vi "Judgment.vi"(7 "Name (\"\" to Use UUID)":string="Judgment") -> ()   [LabVIEW 2025]
doc: "Compact code template used to create a CSM module with a user interface. This template includes a user Event Structure for responding to user actions. The functionality of this template is identical to the CSM User Interface(UI) Module Template VI.\n\n\n> [!NOTE] <b>CSM Naming Rules</b>\n>\n> - CSM module name must be unique. Otherwise, CSM enters a `Critical Error` state.\n> - If the input module name is an empty string (\"\"), the system uses a UUID as the module name. Such a module is marked as standalone mode and does not appear in the module list.\n> - Worker Mode Rule: If the input module name ends with `#`, a worker mode node will be instantiated. Multiple worker mode nodes can form a worker mode module.\n> - Chain of Responsibility Mode Rule: If the input module name ends with `$` followed by a number, a chain of responsibility mode node will be instantiated. Multiple chain of responsibility mode nodes can form a chain of responsibility mode module.\n> - System-Level Module Rule: If the input module name starts with `.`, the module is a system-level module. Under default settings, such modules are not listed by the CSM - List Modules VI and are suitable for instantiating modules that run in the background.\n> - Submodule Rule: `.` is also allowed in a module name to separate the module name into multiple parts. CSM does not have strict rules for submodules. The `.` in the module name only marks the logical relationship between different modules. From an execution perspective, they are considered independent modules. The only difference is that you can obtain a list of logical submodules via the CSM - List Submodules VI.\n\n\n-- <b>Controls</b> --\n- <b>Name (\"\" to use UUID)</b>: CSM module name. Refer to <b>CSM Naming Rules</b> for module naming rules."
uses:
  <userlib>/_NEVSTOP/Communicable State Machine(CSM)/AdvanceAPI/CSM - Revert Arguments-Safe String.vi
  <userlib>/_NEVSTOP/Communicable State Machine(CSM)/_Shared/Trim Single-line Text.vi
  <userlib>/_NEVSTOP/Communicable State Machine(CSM)/AdvanceAPI/CSM - Break Down Multiple States String.vi
  <userlib>/_NEVSTOP/Communicable State Machine(CSM)/AdvanceAPI/CSM - Compact Multiple States.vi
  <userlib>/_NEVSTOP/Communicable State Machine(CSM)/AdvanceAPI/CSM - Make String Arguments Safe.vi
  <userlib>/_NEVSTOP/Communicable State Machine(CSM)/AdvanceAPI/CSM - Keywords.vi
  <userlib>/_NEVSTOP/Communicable State Machine(CSM)/Communicable State Machine.lvlib
panel:
  in  "Array":i32[](array[numeric])
  out "State History":string
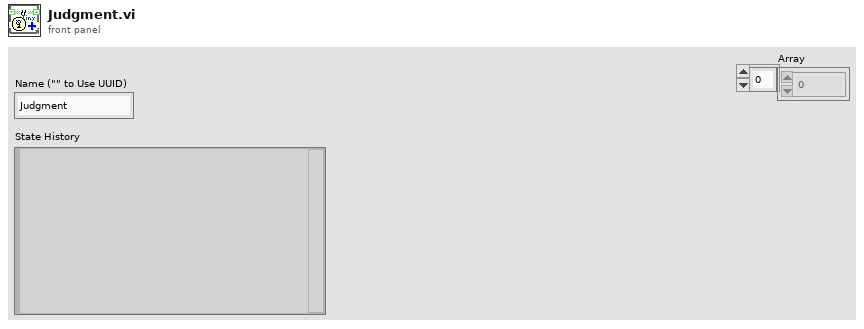
[diagram p1: front panel]
types:
  T1 = enum32{"Invalid", "Standard", "Closed", "Hidden", "Minimized", "Maximized"}
  T2 = enum32{"invalid app kind", "Development System", "Run Time System", "Student Edition", "Embedded LabVIEW", "Evaluation", "Custom"}
  T3 = typedef "Communicable State Machine.lvlib/_CSM_Response Source Message.ctl" = cluster{"‘State":string, "’Arguments":string, "’Error":errorcluster}
  T4 = cluster{"Current VI Reference":refnum<vi>, "Close Panel on Exit?":bool}
  T5 = cluster{"Core":cluster{"Current VI Reference":refnum<vi>, "Close Panel on Exit?":bool}, "T0":i64, "BeatInterval":i32, "NoteIndex":i32}
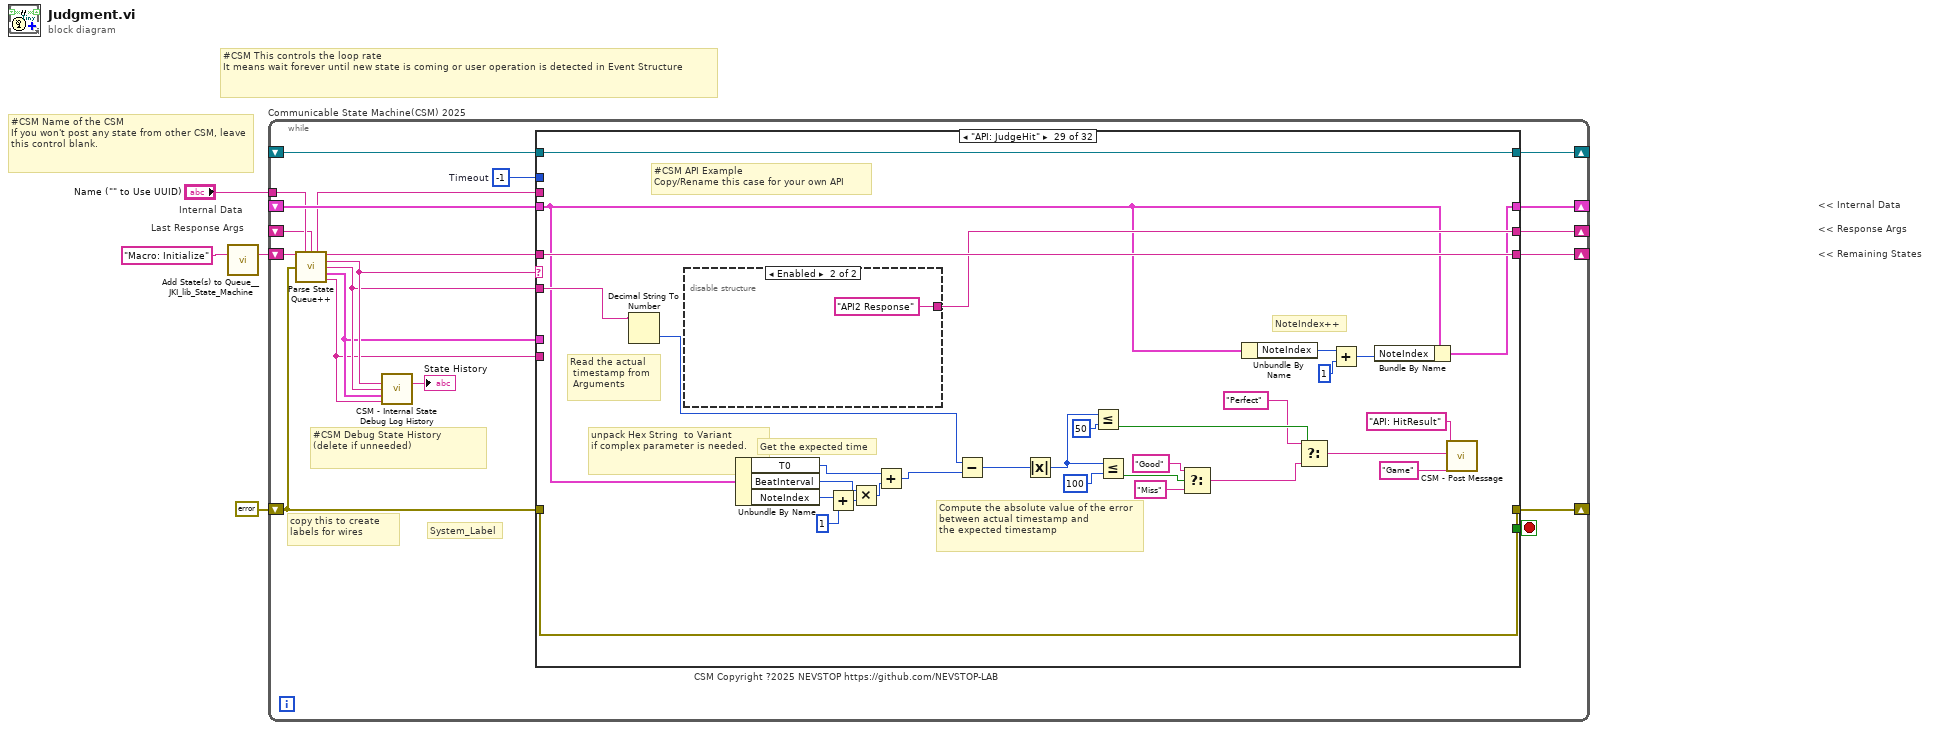
[diagram p0: block diagram]
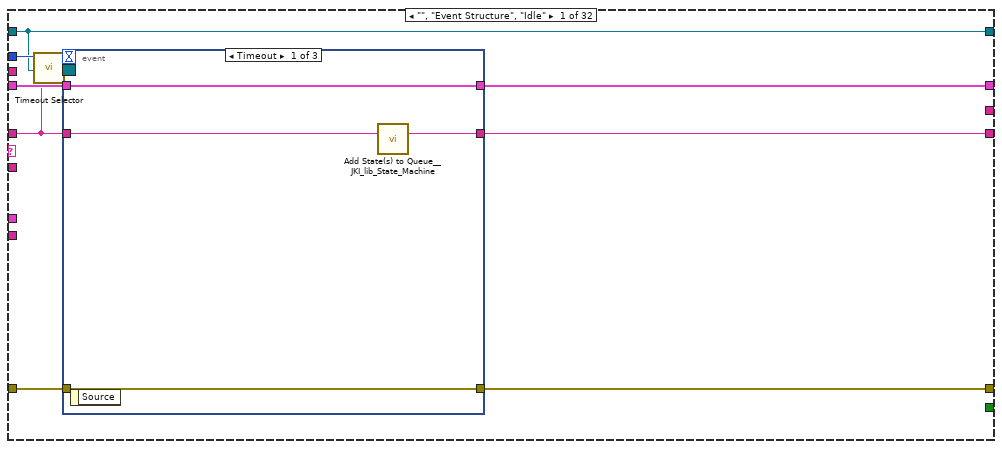
[diagram p2: hidden frame]
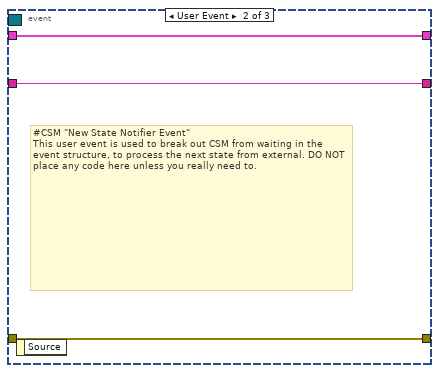
[diagram p3: hidden frame]
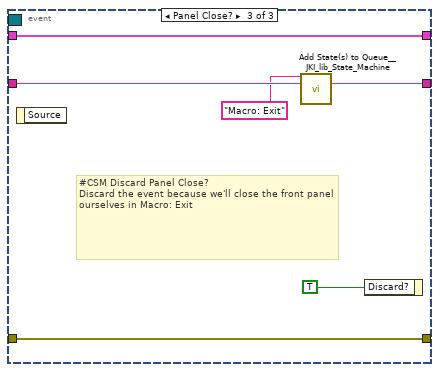
[diagram p4: hidden frame]
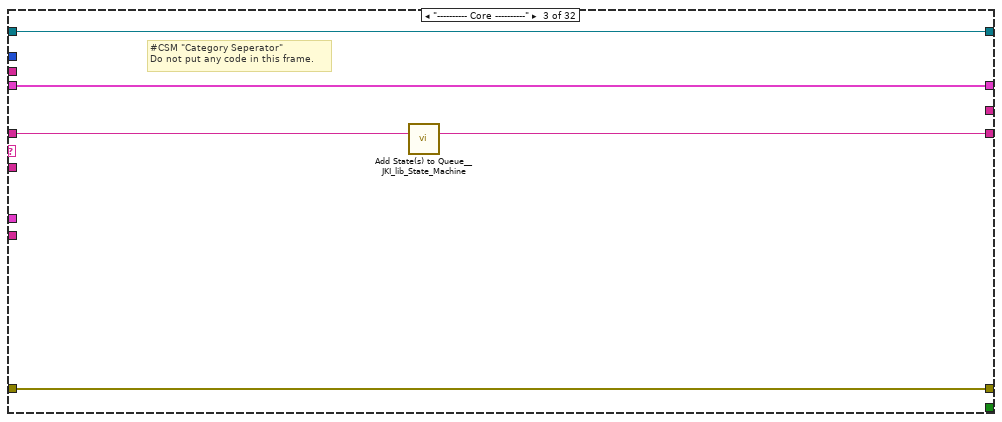
[diagram p6: hidden frame]
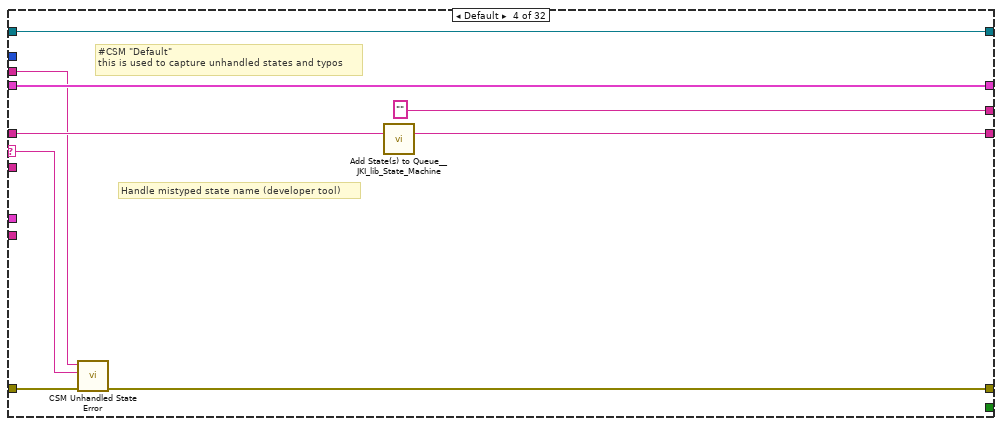
[diagram p7: hidden frame]
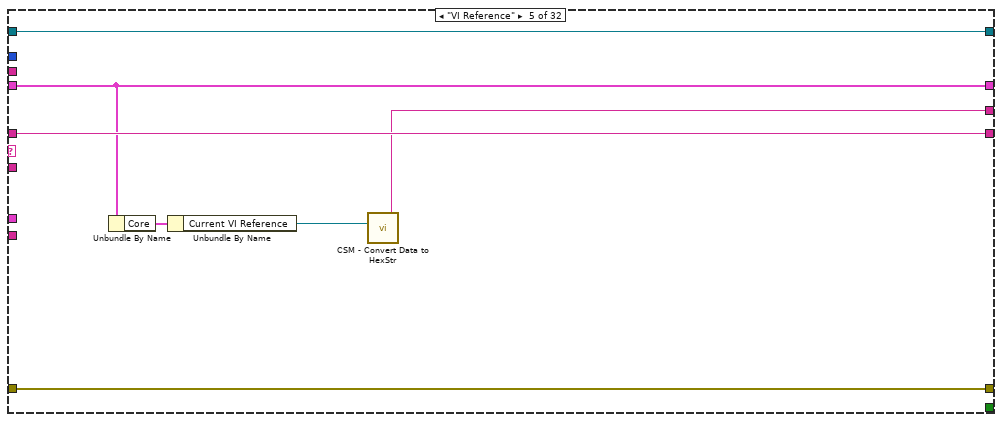
[diagram p8: hidden frame]
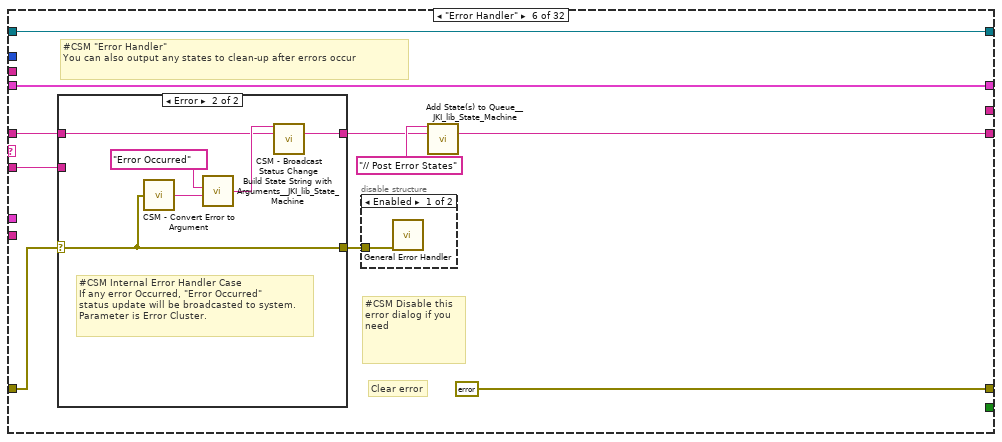
[diagram p9: hidden frame]
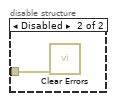
[diagram p10: hidden frame]
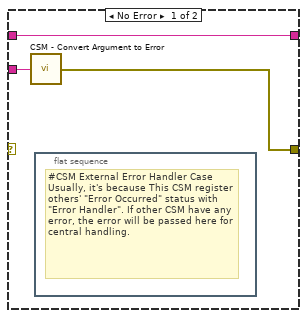
[diagram p11: hidden frame]
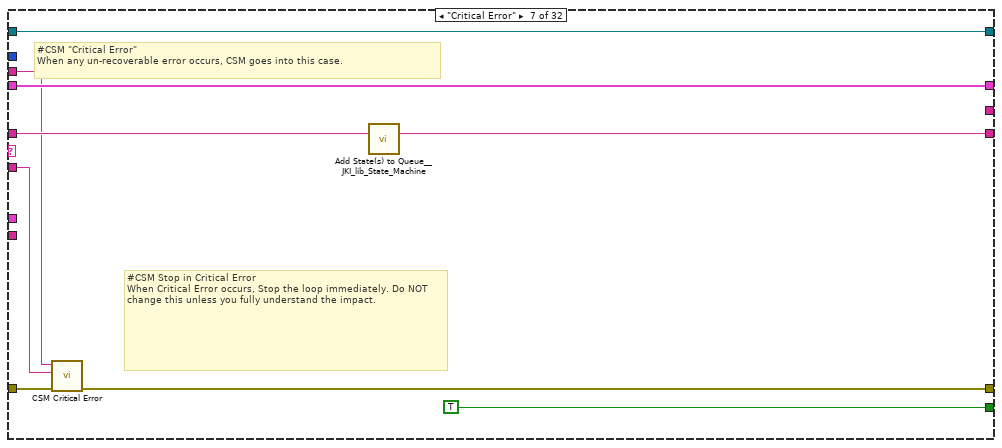
[diagram p12: hidden frame]
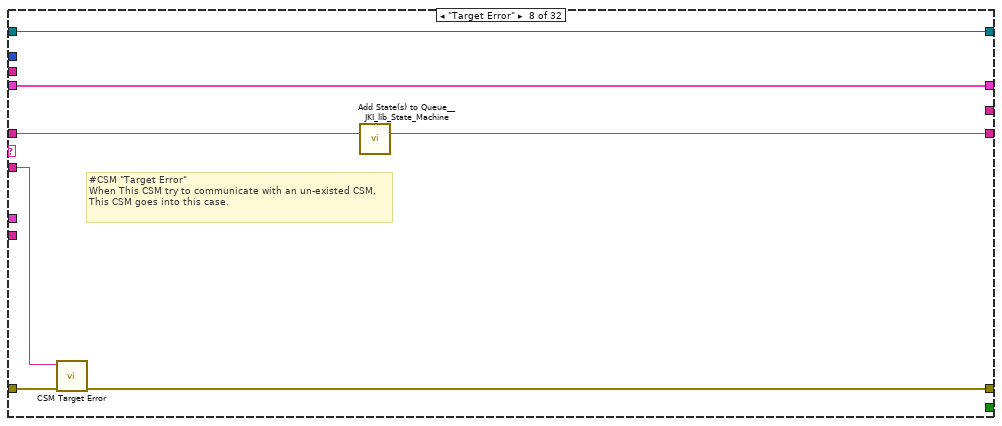
[diagram p13: hidden frame]
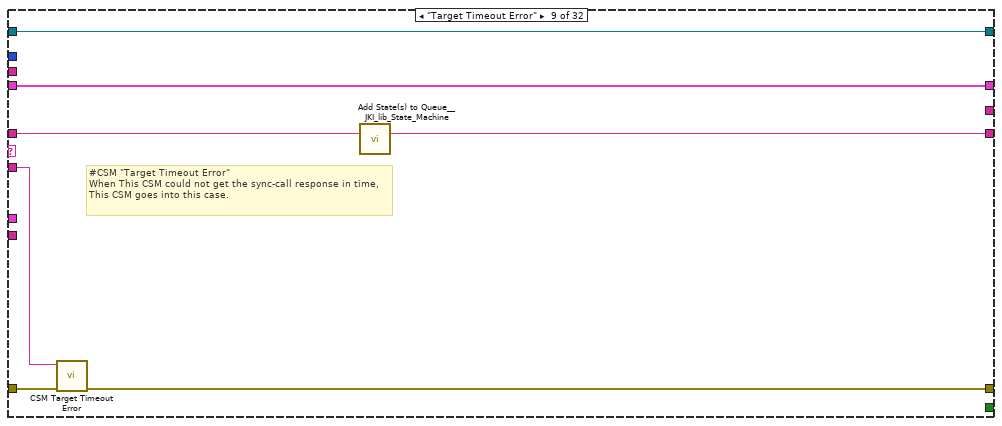
[diagram p14: hidden frame]
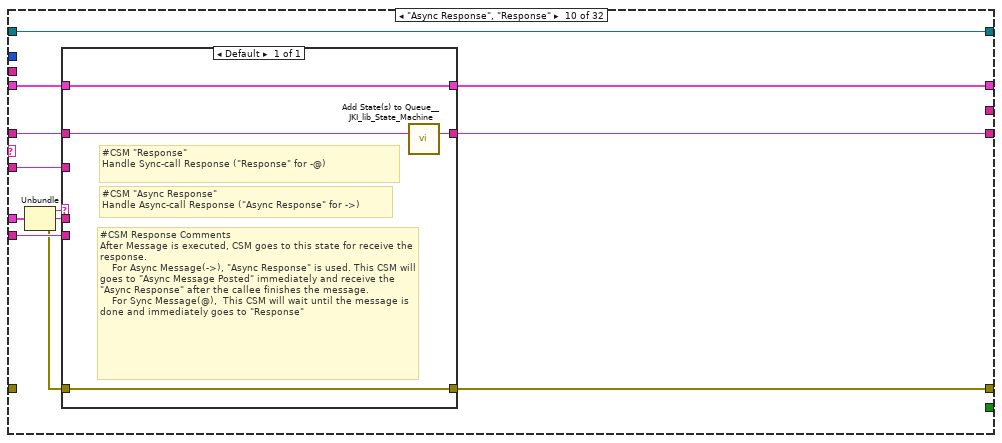
[diagram p15: hidden frame]
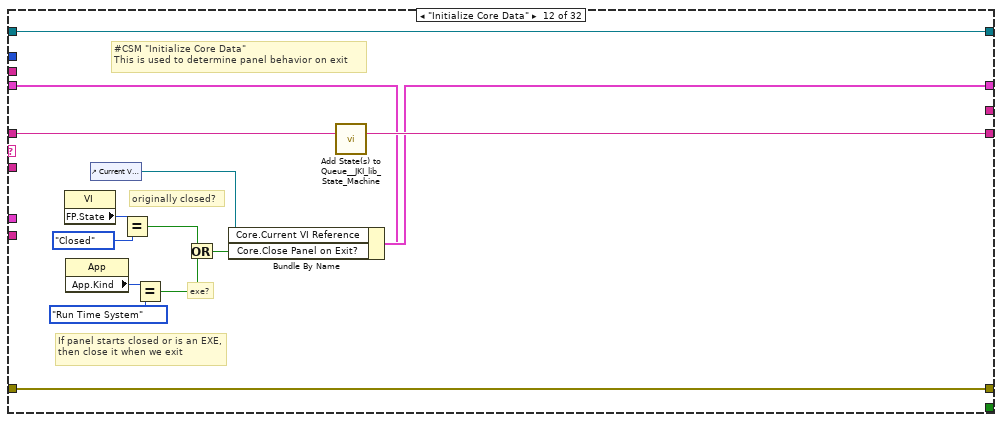
[diagram p17: hidden frame]
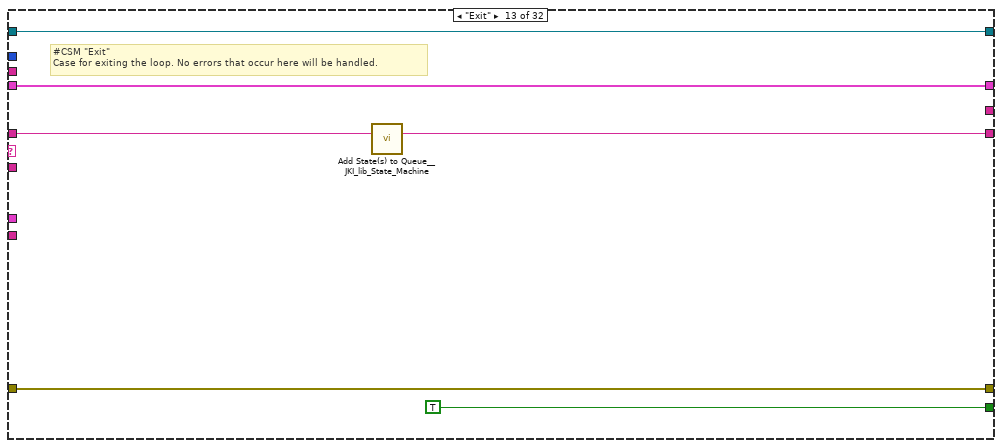
[diagram p18: hidden frame]
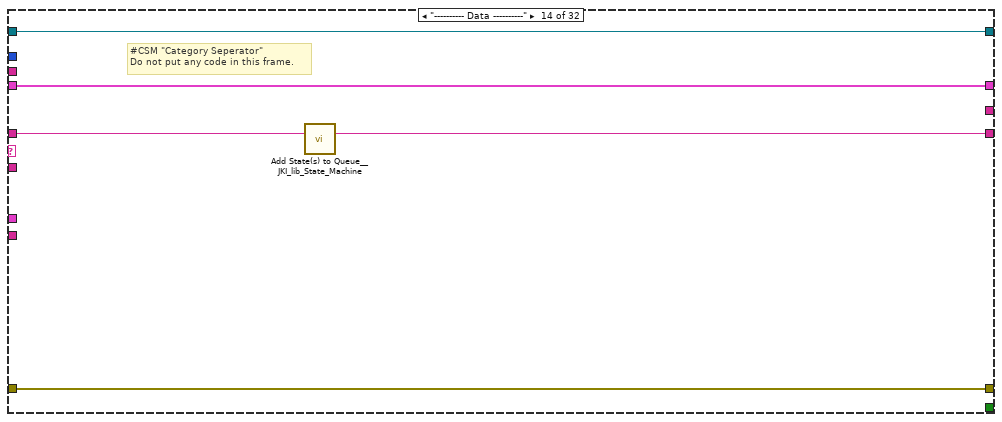
[diagram p19: hidden frame]
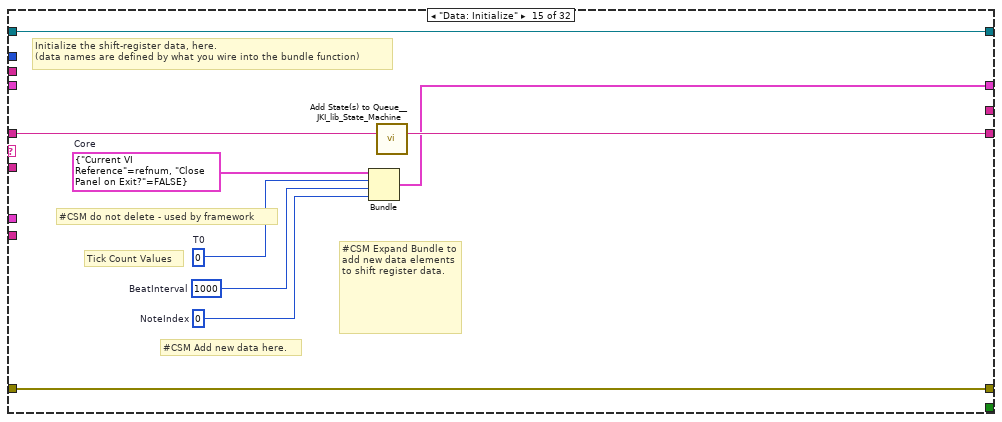
[diagram p20: hidden frame]
diagram:
  # "Last Response Args"
  # "Internal Data"
  # "#CSM Name of the CSM\nIf you won't post any state from other CSM, leave this control blank."
  # "#CSM This controls the loop rate\nIt means wait forever until new state is coming or user operation is detected in Event Structure"
  # "<< Internal Data"
  # "<< Response Args"
  # "<< Remaining States"
  n1 = call <vilib>:"Add State(s) to Queue__JKI_lib_State_Machine.vi"("State(s) in (\"\")"="Macro: Initialize" ("Init State(\"Macro: Initialize\")")) -> ("States Out"=w4:string)  [unwired: 14 in]
  n2 = while "Communicable State Machine(CSM) 2025" {
    shift-right: [w19] -> _
    shift-left: _ -> [w18]
    shift-right: [w22] -> _
    shift-left: errorcluster {"status"=FALSE, "code"=0, "source"=""} ("error out") -> [w16]
    shift-right: [w21] -> _
    shift-left: w4 -> [w23]
    tunnel: "Name (\"\" to Use UUID)" -> [w12]
    shift-right: [w15] -> _
    shift-left: _ -> [w6]
    shift-right: [w14] -> _
    shift-left: _ -> [w13]
    stop <- w20 stop-if-true
    w17 = -1  # Timeout
    # "#CSM Debug State History\n(delete if unneeded)"
    # "copy this to create labels for wires"
    # "System_Label"
    # "CSM Copyright ?2025 NEVSTOP https://github.com/NEVSTOP-LAB"
    n3 = call <userlib>:"Parse State Queue++.vi"("State Queue"=w23, "Name (\"\" to Use UUID)"=w12, "Response Arguments"=w6, "Previous Error"=w16) -> ("Name Used"=w7:string, "Remaining States"=w24:string, "Current State"=w11:string, "Arguments"=w10:string, "Additional Information"=w9:T3, "Source CSM"=w8:string)  [unwired: 6 in]
    n4 = call <userlib>:"CSM - Internal State Debug Log History.vi"("State"=w11, "Arguments (\"\")"=w10, ">> Response Source Message >>"=w9, "Source (\"\")"=w8) -> ("Debug Log"=→"State History":string)  [unwired: 11 in]
    n5 = case shown="\"API: JudgeHit\"" w11 {
      selector: w11 -> [_ _ _ w58 _ _ _ _ _ _ _ _ _ _ _ _ _ _ _ _ _ _ _ _ _ _ _ _ _ _ _ _]
      tunnel: w24 -> [w25 w49 w55 w63 w70 w76 w99 w105 w112 w121 w134 w149 w155 w160 w169 w176 w181 w188 w192 w198 w203 w210 w226 w296 w302 w314 w317 w333 w364 w372 w377 w382]
      tunnel: w10 -> [_ _ _ _ _ w75 w94 w104 w111 w120 _ _ _ _ _ _ _ _ _ _ _ w205 w220 _ _ _ _ w330 w361 _ _ _]
      tunnel: w18 -> [w32 w48 w52 w61 w69 w80 w100 w107 w114 w123 w133 w142 w153 w157 _ w171 w178 w187 w191 w195 w201 w208 w222 w293 w299 w311 w316 w324 w339 w369 w374 w379]
      tunnel: [w31 w50 w53 w56 w71 errorcluster {"status"=FALSE, "code"=0, "source"=""} ("error out") w95 w102 w109 w126 w135 w146 w152 w158 w166 w172 w179 w182 w190 w196 w200 w206 w223 w294 w300 w312 w318 w334 w365 w370 w375 w380] -> w22
      tunnel: w16 -> [w30 w50 w53 w64 w71 w77 w101 w103 w110 _ w135 w146 w152 w158 w166 w173 w179 _ w193 w196 w200 w207 w224 w294 w300 w312 w318 w334 w365 w370 w375 w380]
      tunnel: [w33 w49 w54 w62 w70 w72 w98 w108 w115 w122 w134 w148 w154 w159 w168 w175 w180 w188 w192 w197 w202 w209 w225 w295 w301 w313 w317 w333 w364 w371 w376 w381] -> w21
      tunnel: [_ _ _ _ _ _ TRUE _ _ _ _ _ TRUE _ _ _ _ _ _ _ _ _ _ _ _ _ _ _ _ _ _ _] -> w20
      tunnel: [w29 w48 w52 w61 w69 w80 w100 w107 w114 w124 w133 w147 w153 w157 w167 w171 w178 w187 w191 w195 w201 w208 w222 w293 w299 w311 w316 w320 w338 w369 w374 w379] -> w19
      tunnel: w17 -> [w28 _ _ _ _ _ _ _ _ _ _ _ _ _ _ _ _ _ _ _ _ _ _ _ _ _ _ _ _ _ _ _]
      tunnel: w8 -> [_ _ _ _ _ _ _ _ _ w118 _ _ _ _ _ _ _ _ _ _ _ _ _ _ _ _ _ _ _ _ _ _]
      tunnel: w9 -> [_ _ _ _ _ _ _ _ _ w125 _ _ _ _ _ _ _ _ _ _ _ _ _ _ _ _ _ _ _ _ _ _]
      tunnel: [_ _ _ "" w65 _ _ _ _ _ _ _ _ _ _ _ _ _ _ _ _ _ _ _ _ _ _ "API1 Response" w362 _ _ _] -> w15
      tunnel: [w27 w47 w51 w59 w68 w79 w96 w106 w113 w127 w132 w136 w150 w156 w164 w170 w177 w186 w189 w194 w199 w204 w219 w292 w297 w304 w315 w332 w363 w368 w373 w378] -> w14
      tunnel: w13 -> [w27 w47 w51 w59 w68 w79 w96 w106 w113 w127 w132 w136 w150 w156 w164 w170 w177 _ w189 w194 w199 w204 w219 w292 w297 w304 w315 w332 w363 w368 w373 w378]
      tunnel: w7 -> [_ _ _ w57 _ _ w93 _ _ _ _ _ _ _ _ _ _ w185 _ _ _ _ _ _ _ _ _ _ _ _ _ _]
      frame "", "Event Structure", "Idle" {
        n6 = call <userlib>:"Timeout Selector.vi"("Remaining States"=w25, "Timeout Expected"=w28) -> ("Timeout"=w26:i32)  [unwired: 5 in]
        n7 = event shown="[0] Timeout" {
          selector: w27 -> [_ _ _]
          dyn-events: _ -> [_ _ _]
          timeout: w26 -> [_ _ _]
          tunnel: w25 -> [w37 w39 w46]
          tunnel: [w36 w39 w45] -> w33
          tunnel: w32 -> [w34 w40 w43]
          tunnel: [w35 w38 w44] -> w31
          tunnel: w30 -> [w35 w38 w44]
          tunnel: [w34 w40 w43] -> w29
          event Timeout {
            n8 = event-data() -> ()  [unwired: 1 in, 1 out]
            n9 = call <vilib>:"Add State(s) to Queue__JKI_lib_State_Machine.vi"("State(s) in (\"\")"=w37) -> ("States Out"=w36:string)  [unwired: 14 in]
          }
          event User Event {
            # "#CSM \"New State Notifier Event\"\nThis user event is used to break out CSM from waiting in the event structure, to process the next state from external. DO NOT place any code here unless you really need to."
            n10 = event-data() -> ()  [unwired: 1 in, 1 out]
          }
          event Panel Close? {
            # "#CSM Discard Panel Close?\nDiscard the event because we'll close the front panel ourselves in Macro: Exit"
            n11 = event-data() -> ()  [unwired: 1 in, 1 out]
            n12 = call <vilib>:"Add State(s) to Queue__JKI_lib_State_Machine.vi"("State(s) in Front (\"\")"="Macro: Exit", "State(s) in (\"\")"=w46) -> ("States Out"=w45:string)  [unwired: 13 in]
            n13 = event-data("Discard?"=TRUE) -> ()  [unwired: 1 in, 1 out]
          }
        }
      }
      frame "CSM Documentation" {
        # "#CSM README FIRST\n\nCommunicable State Machine(CSM) is a LabVIEW application framework that builds upon JKI State Machine(JKISM). It follows the pattern of JKISM and extends the keywords to describe message communication between modules, including concepts such as Sync-Message, Async-Message, Subscription/Unsubscription of status - essential elements for creating reusable code modules. For more information, please visit the CSM wiki: https://nevstop-lab.github.io/CSM-Wiki/\n\nFor instructions on JKI State Machine, visit: http://jki.net/state-machine/\nFor information about CSM, visit: https://github.com/NEVSTOP-LAB"
        # "#CSM \"Documentation\"\nCase for holding CSM Documenation"
      }
      frame "---------- Core ----------" {
        # "#CSM \"Category Seperator\"\nDo not put any code in this frame."
        n14 = call <vilib>:"Add State(s) to Queue__JKI_lib_State_Machine.vi"("State(s) in (\"\")"=w55) -> ("States Out"=w54:string)  [unwired: 14 in]
      }
      frame Default {
        # "#CSM \"Default\"\nthis is used to capture unhandled states and typos"
        # "Handle mistyped state name (developer tool)"
        n15 = call <userlib>:"CSM Unhandled State Error.vi"("error in (no error)"=w64, "Undefined State"=w58, "CSM Name"=w57) -> ("error out"=w56:errorcluster)  [unwired: 8 in]
        n16 = call <vilib>:"Add State(s) to Queue__JKI_lib_State_Machine.vi"("State(s) in (\"\")"=w63) -> ("States Out"=w62:string)  [unwired: 14 in]
      }
      frame "VI Reference" {
        n17 = Unbundle By Name(w69) -> ("Core"=w67:T4)
        n18 = Unbundle By Name(w67) -> ("Current VI Reference"=w66:refnum<vi>)
        n19 = call <userlib>:"CSM - Convert Data to HexStr.vi"("Variant"=w66) -> ("HEX String (0-9,A-F)"=w65:string)  [unwired: 8 in]
      }
      frame "Error Handler" {
        # "#CSM Disable this error dialog if you need"
        # "#CSM \"Error Handler\"\nYou can also output any states to clean-up after errors occur"
        # "Clear error"
        n20 = case shown="Error" w77 {
          selector: w77 -> [_ w87]
          tunnel: [w86 w89] -> w73
          tunnel: w76 -> [w86 w88]
          tunnel: w75 -> [w85 _]
          tunnel: [w84 w87] -> w78
          frame No Error {
            n21 = call <userlib>:"CSM - Convert Argument to Error.vi"("Argument"=w85) -> ("Error"=w84:errorcluster)  [unwired: 4 in]
            n22 = flat-sequence {
              frame #0 {
                # "#CSM External Error Handler Case\nUsually, it's because This CSM register others' \"Error Occurred\" status with \"Error Handler\". If other CSM have any error, the error will be passed here for central handling."
              }
            }
          }
          frame Error {
            # "#CSM Internal Error Handler Case \nIf any error Occurred, \"Error Occurred\" \nstatus update will be broadcasted to system.\nParameter is Error Cluster."
            n23 = call <userlib>:"CSM - Convert Error to Argument.vi"("Error"=w87) -> ("Argument"=w91:string)  [unwired: 4 in]
            n24 = call <vilib>:"Build State String with Arguments__JKI_lib_State_Machine.vi"("Arguments (\"\")"=w91, "State"="Error Occurred" ("Status with Arguments")) -> ("State with Arguments"=w90:string)  [unwired: 4 in]
            n25 = call <userlib>:"CSM - Broadcast Status Change.vi"("Status With Arguments"=w90, "State Queue"=w88) -> ("Remaining States"=w89:string)  [unwired: 13 in]
          }
        }
        n26 = disable-structure shown="Enabled" {
          disable-tunnel: w78 -> [w82 w83]
          frame Enabled {
            n27 = call <vilib>:"General Error Handler.vi"("error in (no error)"=w82) -> ()  [unwired: 10 in, 5 out]
          }
          frame Disabled {
            n28 = call <vilib>:"Clear Errors.vi"("error in (no error)"=w83) -> ()  [unwired: 5 in, 2 out]
          }
        }
        n29 = call <vilib>:"Add State(s) to Queue__JKI_lib_State_Machine.vi"("State(s) in Front (\"\")"="// Post Error States", "State(s) in (\"\")"=w73) -> ("States Out"=w72:string)  [unwired: 13 in]
      }
      frame "Critical Error" {
        # "#CSM Stop in Critical Error\nWhen Critical Error occurs, Stop the loop immediately. Do NOT change this unless you fully understand the impact."
        # "#CSM \"Critical Error\"\nWhen any un-recoverable error occurs, CSM goes into this case."
        n30 = call <userlib>:"CSM Critical Error.vi"("error in (no error)"=w101, "Arugments (As Reason)"=w94, "CSM Name"=w93) -> ("error out"=w95:errorcluster)  [unwired: 8 in]
        n31 = call <vilib>:"Add State(s) to Queue__JKI_lib_State_Machine.vi"("State(s) in (\"\")"=w99) -> ("States Out"=w98:string)  [unwired: 14 in]
      }
      frame "Target Error" {
        # "#CSM \"Target Error\"\nWhen This CSM try to communicate with an un-existed CSM, This CSM goes into this case."
        n32 = call <userlib>:"CSM Target Error.vi"("error in (no error)"=w103, "Arguments (As CSM Name)"=w104) -> ("error out"=w102:errorcluster)  [unwired: 9 in]
        n33 = call <vilib>:"Add State(s) to Queue__JKI_lib_State_Machine.vi"("State(s) in (\"\")"=w105) -> ("States Out"=w108:string)  [unwired: 14 in]
      }
      frame "Target Timeout Error" {
        # "#CSM \"Target Timeout Error\"\nWhen This CSM could not get the sync-call response in time, This CSM goes into this case."
        n34 = call <userlib>:"CSM Target Timeout Error.vi"("error in (no error)"=w110, "Arguments (As CSM Name)"=w111) -> ("error out"=w109:errorcluster)  [unwired: 9 in]
        n35 = call <vilib>:"Add State(s) to Queue__JKI_lib_State_Machine.vi"("State(s) in (\"\")"=w112) -> ("States Out"=w115:string)  [unwired: 14 in]
      }
      frame "Async Response", "Response" {
        n36 = Unbundle(w125) -> ("‘State"=w119:string, "’Arguments"=w117:string, "’Error"=w116:errorcluster)
        n37 = case shown="Default" w119 {
          tunnel: [w131] -> w126
          tunnel: w116 -> [w131]
          tunnel: [w130] -> w124
          tunnel: w123 -> [w130]
          tunnel: [w128] -> w122
          tunnel: w121 -> [w129]
          tunnel: w120 -> [_]
          tunnel: w118 -> [_]
          tunnel: w117 -> [_]
          frame Default {
            # "#CSM Response Comments\nAfter Message is executed, CSM goes to this state for receive the response.\n    For Async Message(->), \"Async Response\" is used. This CSM will goes to \"Async Message Posted\" immediately and receive the \"Async Response\" after the callee finishes the message.\n    For Sync Message(@),  This CSM will wait until the message is done and immediately goes to \"Response\""
            # "#CSM \"Async Response\"\nHandle Async-call Response (\"Async Response\" for ->)"
            # "#CSM \"Response\"\nHandle Sync-call Response (\"Response\" for -@)"
            n38 = call <vilib>:"Add State(s) to Queue__JKI_lib_State_Machine.vi"("State(s) in (\"\")"=w129) -> ("States Out"=w128:string)  [unwired: 14 in]
          }
        }
      }
      frame "Async Message Posted" {
        # "#CSM \"Async Message Posted\"\nAfter Async Message is posted (-> or ->| ), CSM goes to this state for post-action.\nYou can use Argument - State to tell which Async Message is called."
      }
      frame "Initialize Core Data" {
        # "#CSM \"Initialize Core Data\"\nThis is used to determine panel behavior on exit"
        # "originally closed?"
        # "exe?"
        # "If panel starts closed or is an EXE, then close it when we exit"
        n39 = property class="VI"() -> ("FP.State"=w139:T1)  [unwired: 2 in, 2 out]
        n40 = property class="App"() -> ("App.Kind"=w145:T2)  [unwired: 2 in, 2 out]
        n41 = control-ref of="Current VI Reference"() -> (w140:refnum<vi>)
        n42 = Equal?(x=w139, y=T1."Closed" ("Front Panel Window:State")) -> (x = y?=w137:bool)
        n43 = Equal?(x=w145, y=T2."Run Time System" ("Application:Kind")) -> (x = y?=w143:bool)
        n44 = Or(x=w137, y=w143) -> (x .or. y?=w141:bool)
        n45 = Bundle By Name(cluster=w142, "Core.Current VI Reference"=w140, "Core.Close Panel on Exit?"=w141) -> (w147:T5)
        n46 = call <vilib>:"Add State(s) to Queue__JKI_lib_State_Machine.vi"("State(s) in (\"\")"=w149) -> ("States Out"=w148:string)  [unwired: 14 in]
      }
      frame "Exit" {
        # "#CSM \"Exit\"\nCase for exiting the loop. No errors that occur here will be handled."
        n47 = call <vilib>:"Add State(s) to Queue__JKI_lib_State_Machine.vi"("State(s) in (\"\")"=w155) -> ("States Out"=w154:string)  [unwired: 14 in]
      }
      frame "---------- Data ----------" {
        # "#CSM \"Category Seperator\"\nDo not put any code in this frame."
        n48 = call <vilib>:"Add State(s) to Queue__JKI_lib_State_Machine.vi"("State(s) in (\"\")"=w160) -> ("States Out"=w159:string)  [unwired: 14 in]
      }
      frame "Data: Initialize" {
        w161 = 0  # NoteIndex
        w162 = 1000  # BeatInterval
        w163 = i64 0  # T0
        w165 = T4 {"Current VI Reference"=refnum, "Close Panel on Exit?"=FALSE}  # Core
        # "Tick Count Values"
        # "#CSM do not delete - used by framework"
        # "#CSM Expand Bundle to add new data elements to shift register data."
        # "#CSM Add new data here."
        # "Initialize the shift-register data, here.\n(data names are defined by what you wire into the bundle function)"
        n49 = Bundle("Core"=w165, "T0"=w163, "BeatInterval"=w162, "NoteIndex"=w161) -> (w167:T5)  [unwired: 1 in]
        n50 = call <vilib>:"Add State(s) to Queue__JKI_lib_State_Machine.vi"("State(s) in (\"\")"=w169) -> ("States Out"=w168:string)  [unwired: 14 in]
      }
      frame "Data: Cleanup" {
        # "Cleanup any data and references, here.\n(this is called automatically, by the Macro: Exit)"
        n51 = Unbundle By Name(w171) -> ("Core.Current VI Reference"=w174:refnum<vi>)
        n52 = Close Reference(reference=w174, error in (no error)=w173) -> (error out=w172:errorcluster)
        n53 = call <vilib>:"Add State(s) to Queue__JKI_lib_State_Machine.vi"("State(s) in (\"\")"=w176) -> ("States Out"=w175:string)  [unwired: 14 in]
      }
      frame "---------- Events ----------" {
        # "#CSM \"Category Seperator\"\nDo not put any code in this frame."
        n54 = call <vilib>:"Add State(s) to Queue__JKI_lib_State_Machine.vi"("State(s) in (\"\")"=w181) -> ("States Out"=w180:string)  [unwired: 14 in]
      }
      frame "Events: Register" {
        # "#CSM \"Events: Register\"\nRegister user event. New Message Event is registered to break CSM waiting in event structure by default."
        # "#CSM Register New Message Event\nRegister message event to break Waiting in Event structure."
        n55 = call <userlib>:"CSM - Get New State Notifier Event.vi"("Name (\"\" to Use UUID)"=w185) -> ("error out"=w183:errorcluster, "New State Notifier Event"=w184:refnum<user-event>)  [unwired: 9 in]
        n56 = register-events(error in=w183, w184) -> (reference out=w186:refnum<event-registration>, error out=w182:errorcluster)  [unwired: 1 in]
      }
      frame "Events: Unregister" {
        # "#CSM \"Events: Unregister\"\nUnregister user event."
        n57 = Unregister For Events(event registration refnum=w189, error in=w193) -> (error out=w190:errorcluster)
      }
      frame "---------- UI ----------" {
        # "#CSM \"Category Seperator\"\nDo not put any code in this frame."
        n58 = call <vilib>:"Add State(s) to Queue__JKI_lib_State_Machine.vi"("State(s) in (\"\")"=w198) -> ("States Out"=w197:string)  [unwired: 14 in]
      }
      frame "UI: Initialize" {
        # "#CSM \"UI: Initialize\"\nInitialize the User Interface, here.\n(this is called automatically, by the Macro: Init)"
        n59 = call <vilib>:"Add State(s) to Queue__JKI_lib_State_Machine.vi"("State(s) in (\"\")"=w203) -> ("States Out"=w202:string)  [unwired: 14 in]
      }
      frame "UI: Cursor Set" {
        # "#CSM \"UI: Cursor Set\"\nSet and Unset Cursor Busy.\n(Usage: \"UI: Cursor Set >> Busy|Idle\")"
        # "Argument"
        n60 = disable-structure shown="Default" {
          disable-tunnel: w207 -> [w213 w218]
          disable-tunnel: [w212 w218] -> w206
          disable-tunnel: w205 -> [w211 _]
          frame condition #0 (active) {
            n61 = case shown="\"Idle\", Default" w211 {
              tunnel: w213 -> [w215 w217]
              tunnel: [w214 w216] -> w212
              frame "Idle", Default {
                n62 = call <vilib>:"Unset Busy.vi"("error in (no error)"=w215) -> ("error out"=w214:errorcluster)  [unwired: 10 in]
              }
              frame "Busy" {
                n63 = call <vilib>:"Set Busy.vi"("error in (no error)"=w217) -> ("error out"=w216:errorcluster)  [unwired: 9 in, 1 out]
              }
            }
          }
          frame condition #1 {
          }
        }
        n64 = call <vilib>:"Add State(s) to Queue__JKI_lib_State_Machine.vi"("State(s) in (\"\")"=w210) -> ("States Out"=w209:string)  [unwired: 14 in]
      }
      frame "UI: Front Panel State" {
        # "#CSM \"UI: Front Panel State\"\nSet Front Panel Open or Closed\n(Usage: \"UI: Front Panel State >> Open|Close\")"
        # "Argument"
        n65 = Unbundle By Name(w222) -> ("Core.Current VI Reference"=w221:refnum<vi>)
        n66 = call <vilib>:"Add State(s) to Queue__JKI_lib_State_Machine.vi"("State(s) in (\"\")"=w226) -> ("States Out"=w225:string)  [unwired: 14 in]
        n67 = case shown="\"Close\", \"Closed\"" w220 {
          tunnel: w224 -> [w232 w247 w258 w271 w284]
          tunnel: [w234 w248 w260 w273 w286] -> w223
          tunnel: w221 -> [w233 w245 w259 w272 w285]
          frame "Open", "Standard", Default {
            w227 = T1."Standard" ("State")
            n68 = property class="VI"(reference=w233, error in=w232) -> (reference out=w230:refnum<vi>, error out=w231:errorcluster, "FP.State"=w229:T1)
            n69 = Not Equal?(x=w229, y=w227) -> (x != y?=w228:bool)
            n70 = case shown="True" w228 {
              tunnel: [w238 w240] -> w234
              tunnel: w231 -> [w237 w240]
              tunnel: w230 -> [w236 _]
              tunnel: w227 -> [w235 _]
              frame True {
                n71 = invoke class="VI" method="FP.Open"(reference=w236, error in=w237, "Activate"=TRUE, "State"=w235) -> (error out=w238:errorcluster)  [unwired: 1 in, 4 out]
              }
              frame False {
              }
            }
          }
          frame "Close", "Closed" {
            n72 = property class="VI"(reference=w245, error in=w247) -> (reference out=w244:refnum<vi>, error out=w246:errorcluster, "FP.State"=w242:T1)
            n73 = Not Equal?(x=w242, y=T1."Closed" ("Front Panel Window:State")) -> (x != y?=w241:bool)
            n74 = case shown="False" w241 {
              tunnel: [w249 w252] -> w248
              tunnel: w246 -> [w249 w251]
              tunnel: w244 -> [_ w250]
              frame False {
              }
              frame True {
                n75 = invoke class="VI" method="FP.Close"(reference=w250, error in=w251) -> (error out=w252:errorcluster)  [unwired: 1 in, 2 out]
              }
            }
          }
          frame "Hidden", "Hide" {
            w253 = T1."Hidden" ("State")
            n76 = property class="VI"(reference=w259, error in=w258) -> (reference out=w256:refnum<vi>, error out=w257:errorcluster, "FP.State"=w255:T1)
            n77 = Not Equal?(x=w255, y=w253) -> (x != y?=w254:bool)
            n78 = case shown="True" w254 {
              tunnel: [w264 w265] -> w260
              tunnel: w257 -> [w263 w265]
              tunnel: w256 -> [w262 _]
              tunnel: w253 -> [w261 _]
              frame True {
                n79 = invoke class="VI" method="FP.Open"(reference=w262, error in=w263, "State"=w261) -> (error out=w264:errorcluster)  [unwired: 2 in, 4 out]
              }
              frame False {
              }
            }
          }
          frame "Minimize", "Minimized" {
            w266 = T1."Minimized" ("State")
            n80 = property class="VI"(reference=w272, error in=w271) -> (reference out=w269:refnum<vi>, error out=w270:errorcluster, "FP.State"=w268:T1)
            n81 = Not Equal?(x=w268, y=w266) -> (x != y?=w267:bool)
            n82 = case shown="True" w267 {
              tunnel: [w277 w278] -> w273
              tunnel: w270 -> [w276 w278]
              tunnel: w269 -> [w275 _]
              tunnel: w266 -> [w274 _]
              frame True {
                n83 = invoke class="VI" method="FP.Open"(reference=w275, error in=w276, "State"=w274) -> (error out=w277:errorcluster)  [unwired: 2 in, 4 out]
              }
              frame False {
              }
            }
          }
          frame "Maximize", "Maximized" {
            w279 = T1."Maximized" ("State")
            n84 = property class="VI"(reference=w285, error in=w284) -> (reference out=w282:refnum<vi>, error out=w283:errorcluster, "FP.State"=w281:T1)
            n85 = Not Equal?(x=w281, y=w279) -> (x != y?=w280:bool)
            n86 = case shown="True" w280 {
              tunnel: [w290 w291] -> w286
              tunnel: w283 -> [w289 w291]
              tunnel: w282 -> [w288 _]
              tunnel: w279 -> [w287 _]
              frame True {
                n87 = invoke class="VI" method="FP.Open"(reference=w288, error in=w289, "State"=w287) -> (error out=w290:errorcluster)  [unwired: 2 in, 4 out]
              }
              frame False {
              }
            }
          }
        }
      }
      frame "---------- Macro ----------" {
        # "#CSM \"Category Seperator\"\nDo not put any code in this frame."
        n88 = call <vilib>:"Add State(s) to Queue__JKI_lib_State_Machine.vi"("State(s) in (\"\")"=w296) -> ("States Out"=w295:string)  [unwired: 14 in]
      }
      frame "Macro: Initialize" {
        w298 = "Data: Initialize\nInitialize Core Data\nEvents: Register\nUI: Initialize\nUI: Front Panel State >> Open"  # Data: Initialize Initialize Core Data Events: Register UI: Initialize UI: Front Panel State >> Open
        # "#CSM \"Macro: Initialize\"\nInitialization Macro (This is called once, when the VI starts)"
        n89 = call <vilib>:"Add State(s) to Queue__JKI_lib_State_Machine.vi"("State(s) in Front (\"\")"=w298, "State(s) in (\"\")"=w302) -> ("States Out"=w301:string)  [unwired: 13 in]
      }
      frame "Macro: Exit" {
        # "#CSM \"Macro: Exit\"\nExit Macro (This is called once, when the VI exits)"
        n90 = Unbundle By Name(w311) -> ("Core.Close Panel on Exit?"=w310:bool)
        n91 = Select(t="UI: Front Panel State >> Close", s=w310, f="") -> (s? t:f=w307:string)
        n92 = call <vilib>:"Add State(s) to Queue__JKI_lib_State_Machine.vi"("State(s) in Front (\"\")"="//Exit Sub-Modules ", "State(s) in (\"\")"=w307, "State(s) at Back (\"\")"="Data: Cleanup\nEvents: Unregister\nExit") -> ("States Out"=w305:string)  [unwired: 12 in]
        n93 = call <vilib>:"Add State(s) to Queue__JKI_lib_State_Machine.vi"("State(s) in Front (\"\")"=w305, "State(s) in (\"\")"=w314) -> ("States Out"=w313:string)  [unwired: 13 in]
      }
      frame "---------- API ----------" {
        # "#CSM \"Category Seperator\"\nDo not put any code in this frame."
      }
      frame "API: BeginInput" {
        # "Reset NoteIndex"
        # "Get T0 and BeatInterval by setting up\n element index as 0 and 1"
        # "#CSM API Example\nCopy/Rename this case for your own API"
        # "#CSM >> Source CSM >>\nIf you need to tell who triggered this state , use this string. If it's this case itself, this string is \"\"."
        # "#CSM >> Arguments >>\nDeal with the parameter if any"
        n94 = Spreadsheet String To Array(delimiter (Tab)=",", format string="%d", spreadsheet string=w330, array type (2D Dbl)="Array") -> (array=w327:i32[])
        n95 = Index Array(array=w327, index #1=0 ("index"), index #2=1 ("index")) -> (element #1=w323:i32, element #2=w322:i32)
        n96 = Bundle By Name(cluster=w324, "T0"=w323, "BeatInterval"=w322, "NoteIndex"=0) -> (w320:T5)
      }
      frame "API: JudgeHit" {
        # "NoteIndex++"
        # "Compute the absolute value of the error between actual timestamp and \nthe expected timestamp"
        # "Get the expected time"
        # "Read the actual\n timestamp from\n Arguments"
        # "#CSM API Example\nCopy/Rename this case for your own API"
        # "unpack Hex String  to Variant\nif complex parameter is needed."
        n97 = Decimal String To Number(string=w361) -> (number=w356:i32)  [unwired: 2 in, 1 out]
        n98 = disable-structure shown="Enabled" {
          disable-tunnel: [w366 "API2 Response"] -> w362
          frame Disabled {
            # "pack variant to hexstr \nif complex response is needed."
            # "complex Response"
            n99 = call <userlib>:"CSM - Convert Data to HexStr.vi"() -> ("HEX String (0-9,A-F)"=w366:string)  [unwired: 9 in]
          }
          frame Enabled {
          }
        }
        n100 = Unbundle By Name(w339) -> ("T0"=w358:i64, "BeatInterval"=w359:i32, "NoteIndex"=w336:i32)
        n101 = Add(x=w336, y=1) -> (x+y=w337:i32)
        n102 = Multiply(x=w359, y=w337) -> (x*y=w360:i32)
        n103 = Add(x=w358, y=w360) -> (x+y=w357:i64)
        n104 = Subtract(x=w356, y=w357) -> (x-y=w355:i64)
        n105 = Absolute Value(x=w355) -> (abs(x)=w353:i64)
        n106 = Less Or Equal?(x=w353, y=i64 50) -> (x <= y?=w351:bool)
        n107 = Less Or Equal?(x=w353, y=i64 100) -> (x <= y?=w349:bool)
        n108 = Select(t="Good", s=w349, f="Miss") -> (s? t:f=w346:string)
        n109 = Unbundle By Name(w339) -> ("NoteIndex"=w341:i32)
        n110 = Select(t="Perfect", s=w351, f=w346) -> (s? t:f=w345:string)
        n111 = Add(x=w341, y=1) -> (x+y=w342:i32)
        n112 = Bundle By Name(cluster=w339, "NoteIndex"=w342) -> (w338:T5)
        n113 = call <userlib>:"CSM - Post Message.vi"("Target Module"="Game", "Arguments (\"\")"=w345, "State"="API: HitResult") -> ()  [unwired: 8 in, 1 out]
      }
      frame "---------- Action ----------" {
        # "#CSM \"Category Seperator\"\nDo not put any code in this frame."
        n114 = call <vilib>:"Add State(s) to Queue__JKI_lib_State_Machine.vi"("State(s) in (\"\")"=w372) -> ("States Out"=w371:string)  [unwired: 14 in]
      }
      frame "Action: action1" {
        # "#CSM \"Internal State\"\nThis category is used for holding internal states"
        n115 = call <vilib>:"Add State(s) to Queue__JKI_lib_State_Machine.vi"("State(s) in (\"\")"=w377) -> ("States Out"=w376:string)  [unwired: 14 in]
      }
      frame "Action: action2" {
        # "#CSM \"Internal State\"\nThis category is used for holding internal states"
        n116 = call <vilib>:"Add State(s) to Queue__JKI_lib_State_Machine.vi"("State(s) in (\"\")"=w382) -> ("States Out"=w381:string)  [unwired: 14 in]
      }
    }
  }
